vi "ECC_v2.vi"() -> ()   [LabVIEW 2013]
uses:
  state_machine.ctl
  <vilib>/DAQmx/write.llb/DAQmx Write (Analog Wfm 1Chan NSamp).vi
  <vilib>/DAQmx/create/channels.llb/DAQmx Create Channel (AO-Voltage-Basic).vi
  <vilib>/DAQmx/configure/timing.llb/DAQmx Timing (Use Waveform).vi
  <vilib>/DAQmx/miscellaneous.llb/DAQmx Fill In Error Info.vi
panel:
  out "AMP_status":bool
  in  "APS/APM":bool
  in  "AMP address":tag="Dev1/port0/line0"
  in  "R&S/5181":bool=TRUE
  out "Pause, s":i32
  out "APS_off_status":bool=TRUE
  out "R&S_off_status":bool=TRUE
  out "Countdown":u32
  in  "Rep_delay":u32
  in  "Finite/Continuous":bool
  in  "ResumeSweep":bool
  in  "PauseSweep":bool
  in  "RF_off_rep":bool
  in  "RF_off_set":bool
  in  "RF_off_cycle":bool
  in  "APS_off_rep":bool=TRUE
  in  "APS_off_set":bool
  in  "APS_off_cycle":bool
  in  "AbortSweep":bool
  in  "Check APS":bool
  in  "ON/OFF_APS":bool
  in  "Check R&S":bool
  in  "ON/OFF_RF":bool
  in  "Use_APS":bool=TRUE
  out "DAC_status":bool
  out "RF_status":bool
  out "i_Current_repetition":i32
  out "N_Cycles_Created":i32
  out "i_Current_cycle":i32
  in  "M_repetitions":i32 min=0
  in  "Set_of_Cycles":T1(array[cluster])=[{"On/Off"=TRUE, "f0, MHz"=32.5, "fm, kHz"=100, "A, mV"=20, "Waveform"=enum."triangle", "N_steps"=500, "T_sweep, s"=0.1, "N_sweeps"=5, "End_Wait, s"=0}] {"End_Wait, s" step=1; "N_sweeps" min=0 step=1; "T_sweep, s" min=0.0 step=0.001 format="%#_6f"; "N_steps" min=0 step=1; "fm, kHz" step=1; "f0, MHz" min=0.0 step=0.001 format="%#_6f"}
  out "APS_status":bool
  in  "APS address":refnum<visa-resource-name>="COM3"
  in  "Init Devices":bool
  in  "Do Sweep":bool
  in  "Exit":bool
  in  "DAC channel":tag="Dev1/ao0"
  in  "RF address":string(combo)="19"
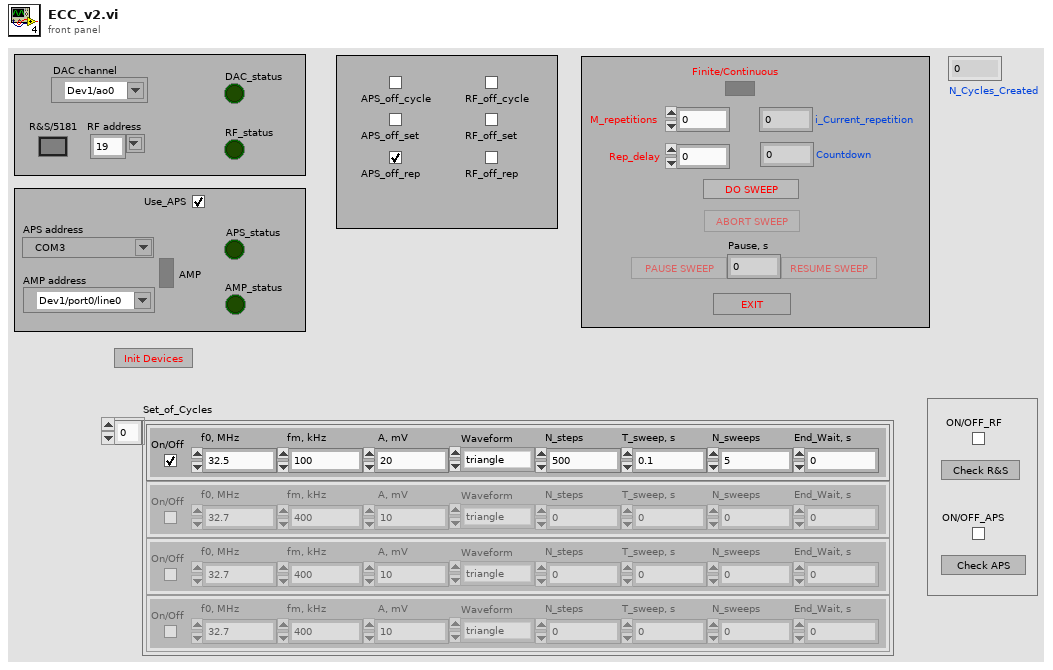
[diagram p1: front panel]
types:
  T1 = cluster{"On/Off":bool, "f0, MHz":dbl, "fm, kHz":i32, "A, mV":i32, "Waveform":enum16{"triangle", "saw_direct", "saw_invert", "sine"}, "N_steps":i32, "T_sweep, s":dbl, "N_sweeps":i32, "End_Wait, s":u32}[]
  T2 = typedef "state_machine.ctl" = enum16{"idle", "init_daq", "init_rf", "init_ps", "cycle_start", "get_wf", "rf_on", "rf_off", "rf_set", "ps_on", "ps_off", "daq_start", "daq_stop", "daq_wait", "daq_dt", "daq_v", "delay", "cycle_reset", "exit", "repetition_reset"}
  T3 = enum8{"Enabled", "Disabled", "Disabled and Grayed Out"}
  T4 = cluster{"On/Off":bool, "f0, MHz":dbl, "fm, kHz":i32, "A, mV":i32, "Waveform":enum16{"triangle", "saw_direct", "saw_invert", "sine"}, "N_steps":i32, "T_sweep, s":dbl, "N_sweeps":i32, "End_Wait, s":u32}
  T5 = enum16{"triangle", "saw_direct", "saw_invert", "sine"}
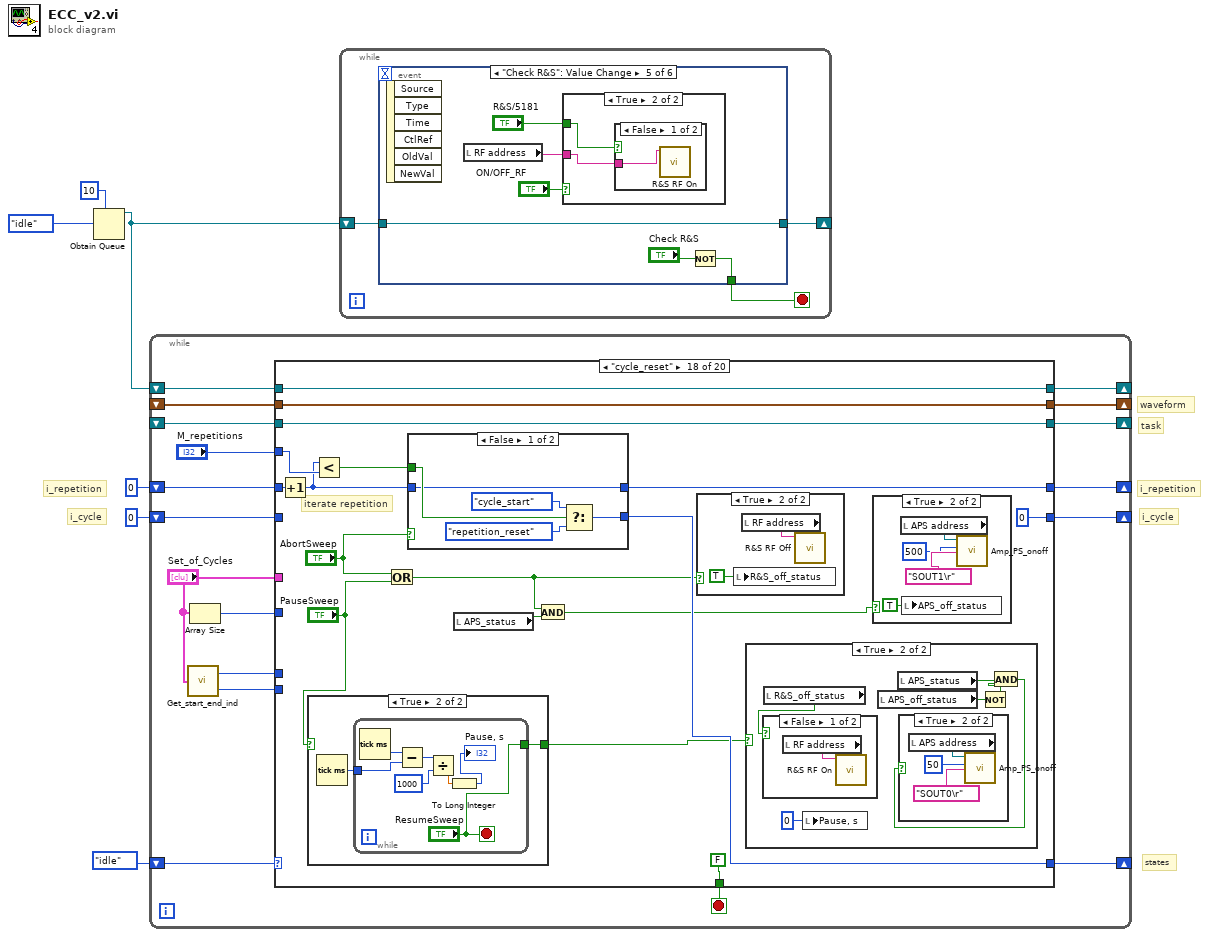
[diagram p0: block diagram]
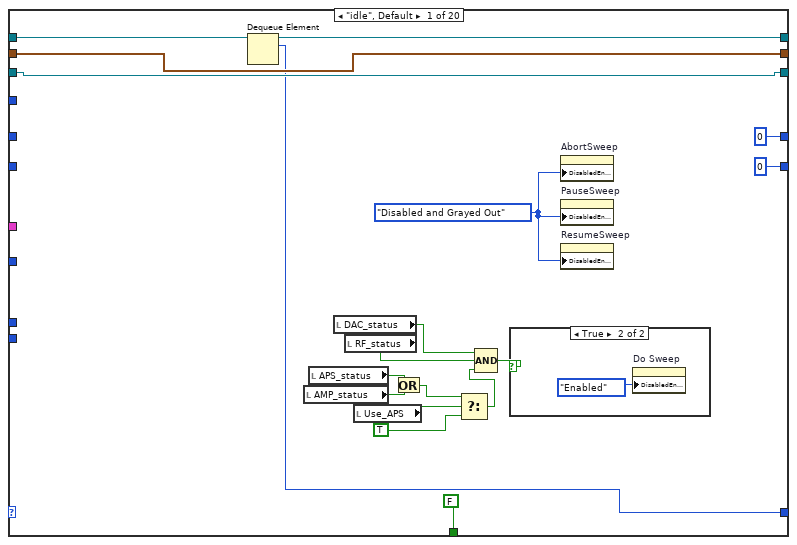
[diagram p2: hidden frame]
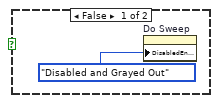
[diagram p3: hidden frame]
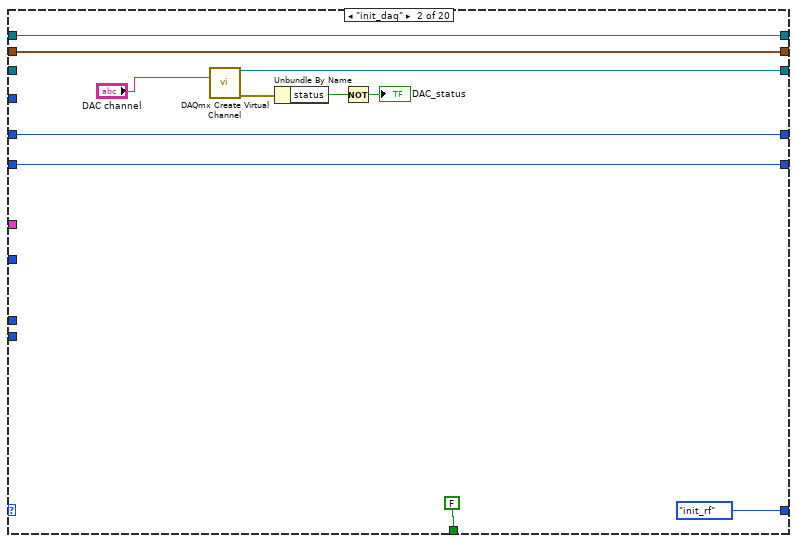
[diagram p4: hidden frame]
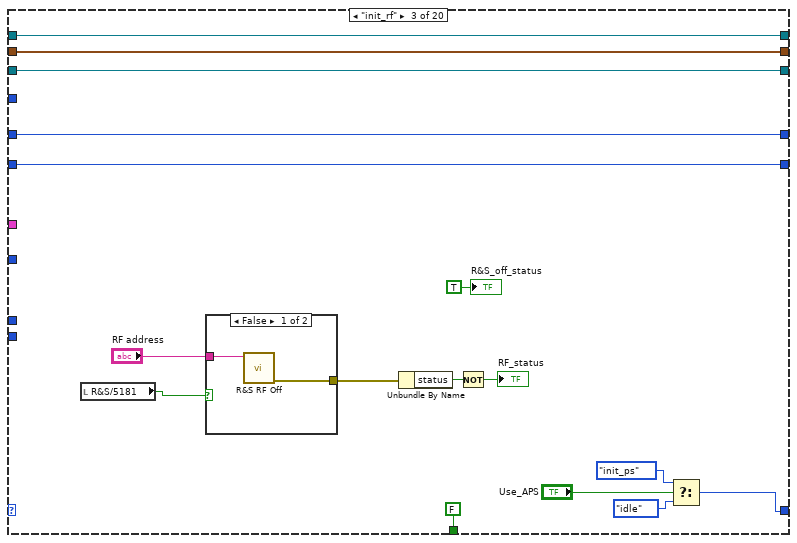
[diagram p5: hidden frame]
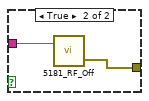
[diagram p6: hidden frame]
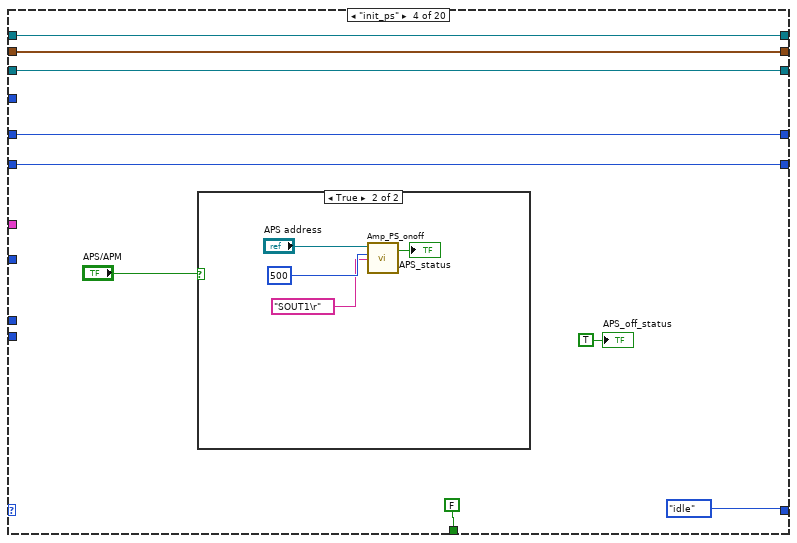
[diagram p7: hidden frame]
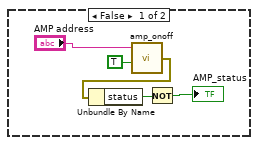
[diagram p8: hidden frame]
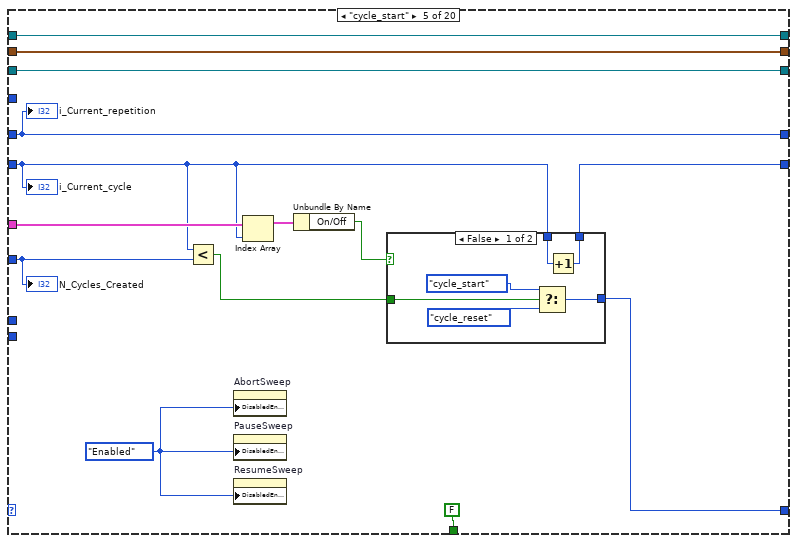
[diagram p9: hidden frame]
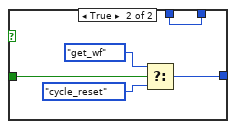
[diagram p10: hidden frame]
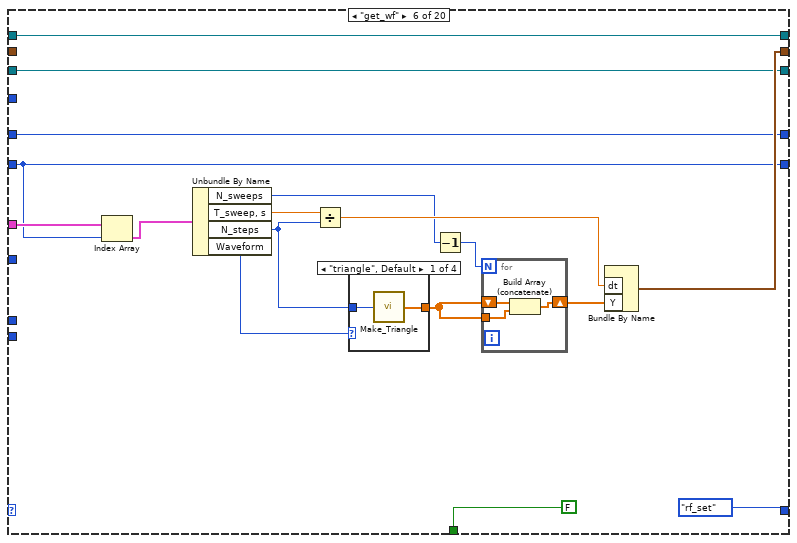
[diagram p11: hidden frame]
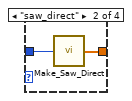
[diagram p12: hidden frame]
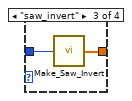
[diagram p13: hidden frame]
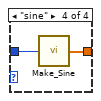
[diagram p14: hidden frame]
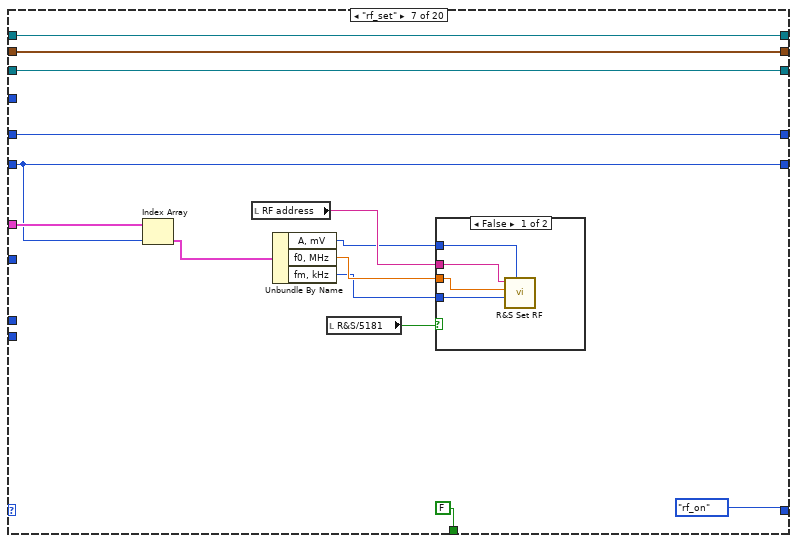
[diagram p15: hidden frame]
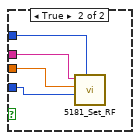
[diagram p16: hidden frame]
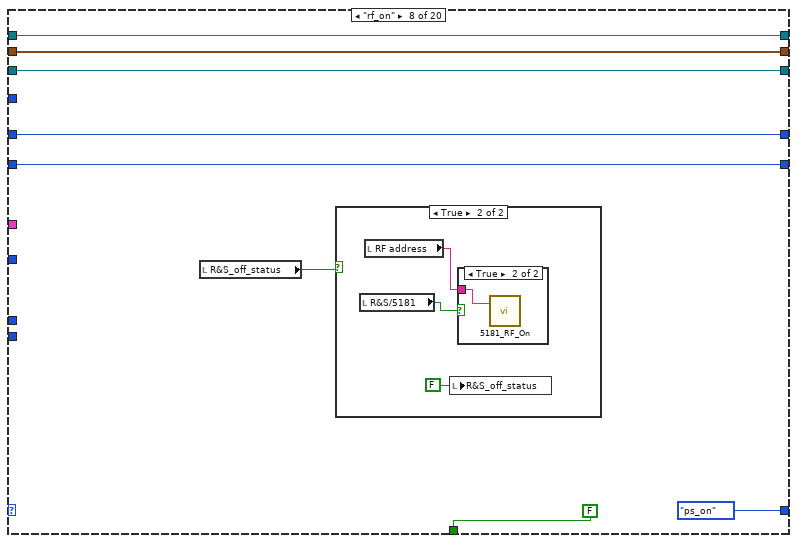
[diagram p17: hidden frame]
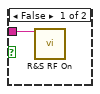
[diagram p19: hidden frame]
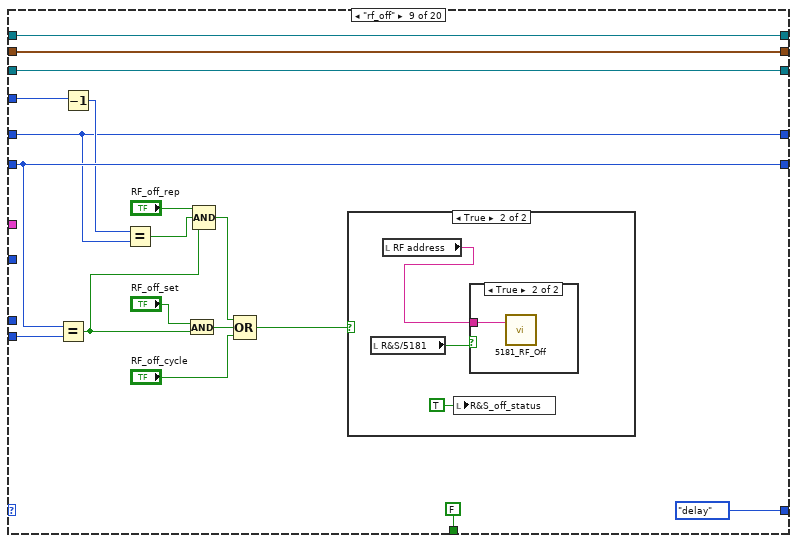
[diagram p20: hidden frame]
diagram:
  # "i_repetition"
  # "i_cycle"
  # "i_repetition"
  # "i_cycle"
  # "states"
  # "waveform"
  # "task"
  n1 = Obtain Queue(max queue size (-1, unlimited)=10, element data type=state_machine."idle") -> (queue out=w4:refnum<queue>)  [unwired: 3 in, 2 out]
  n2 = while {
    shift-right: [w19] -> _
    shift-left: state_machine."idle" -> [w24]
    shift-right: [w23] -> _
    shift-left: _ -> [w21]
    shift-right: [w22] -> _
    shift-left: _ -> [w20]
    shift-right: [w17] -> _
    shift-left: w4 -> [w18]
    shift-right: [w15] -> _
    shift-left: 0 -> [w14]
    shift-right: [w13] -> _
    shift-left: 0 -> [w12]
    stop <- w16 stop-if-true
    n3 = call "Get_start_end_ind.vi"("Set_of_Cycles"="Set_of_Cycles") -> ("start_ind"=w9:i32, "end_ind"=w8:i32)
    n4 = Array Size(array="Set_of_Cycles") -> (size(s)=w11:i32)
    n5 = case shown="\"cycle_reset\"" w24 {
      selector: w24 -> [_ _ _ _ _ _ _ _ _ _ _ _ _ _ _ _ _ _ w376 _]
      tunnel: [w42 w54 w71 w84 w97 w128 w157 w174 w197 w216 w237 w264 w272 w280 w289 w296 w308 w326 w373 w384] -> w23
      tunnel: "Set_of_Cycles" -> [_ _ _ _ w107 w135 w159 _ _ _ _ _ _ _ _ _ w305 _ _ _]
      tunnel: [w41 w53 w70 w83 w98 w129 w156 w175 w198 w215 w236 w263 w271 w279 w288 w297 w309 w325 w372 w385] -> w22
      tunnel: w21 -> [w42 _ w71 w84 w97 w128 w157 w174 w197 w216 w237 w265 w273 w281 w290 w298 w308 w326 w373 w384]
      tunnel: w20 -> [w41 w53 w70 w83 w98 _ w156 w175 w198 w215 w236 w263 w271 w279 w288 w297 w309 w325 w372 w385]
      tunnel: [w38 state_machine."init_rf" w61 state_machine."idle" w103 state_machine."rf_set" state_machine."rf_on" state_machine."ps_on" state_machine."delay" state_machine."daq_dt" state_machine."rf_off" state_machine."daq_wait" state_machine."ps_off" state_machine."daq_stop" state_machine."daq_v" state_machine."daq_start" state_machine."cycle_start" w324 w376 w380] -> w19
      tunnel: w18 -> [w40 w50 w68 w80 w96 w126 w154 w176 w199 w212 w233 w260 w268 w276 w284 w293 w310 w327 w375 w387]
      tunnel: [w39 w50 w68 w80 w96 w126 w154 w176 w199 w212 w233 w260 w268 w276 w284 w293 w310 w327 w375 w387] -> w17
      tunnel: [FALSE FALSE FALSE FALSE FALSE FALSE FALSE FALSE FALSE FALSE FALSE FALSE FALSE FALSE FALSE FALSE FALSE FALSE TRUE FALSE] -> w16
      tunnel: w11 -> [_ _ _ _ w99 _ _ _ _ _ _ _ _ _ _ _ _ _ _ _]
      tunnel: [0 w49 w67 w79 w102 w119 w152 w170 w193 w210 w231 w259 w267 w275 w283 w292 w300 0 w371 w386] -> w15
      tunnel: w14 -> [_ w49 w67 w79 w100 w119 w152 w170 w193 w210 w231 w259 w267 w275 w283 w292 w299 _ w371 w386]
      tunnel: [0 w48 w66 w78 w95 w121 w153 w173 w185 w211 w227 w258 w266 w274 w282 w291 w307 w321 w370 0] -> w13
      tunnel: w12 -> [_ w48 w66 w78 w95 w121 w153 w173 w185 w211 w227 w258 w266 w274 w282 w291 w307 w322 w370 _]
      tunnel: "M_repetitions" -> [_ _ _ _ _ _ _ _ w190 _ w229 _ _ _ _ _ _ w329 _ _]
      tunnel: w9 -> [_ _ _ _ _ _ _ _ _ _ _ _ _ _ _ _ _ _ _ _]
      tunnel: w8 -> [_ _ _ _ _ _ _ _ w194 _ w232 _ _ _ _ _ _ _ _ _]
      frame "idle", Default {
        w28 = T3."Disabled and Grayed Out" ("Disabled")
        n6 = Dequeue Element(queue=w40) -> (queue out=w39:refnum<queue>, element=w38:T2)  [unwired: 2 in, 2 out]
        n7 = local read "AMP_status"() -> (w26:bool)
        n8 = local read "APS_status"() -> (w27:bool)
        n9 = local read "DAC_status"() -> (w34:bool)
        n10 = local read "RF_status"() -> (w33:bool)
        n11 = local read "Use_APS"() -> (w32:bool)
        n12 = Or(x=w27, y=w26) -> (x .or. y?=w25:bool)
        n13 = Select(t=w25, s=w32, f=TRUE) -> (s? t:f=w30:bool)
        n14 = Compound Arithmetic op=AND(w34, w33, w30) -> (w29:bool)
        n15 = case shown="True" w29 {
          frame False {
            n16 = property on="Do Sweep" class="Bool"("DisabledEnum"=T3."Disabled and Grayed Out" ("Disabled")) -> ()  [unwired: 2 in, 2 out]
          }
          frame True {
            n17 = property on="Do Sweep" class="Bool"("DisabledEnum"=T3."Enabled" ("Disabled")) -> ()  [unwired: 2 in, 2 out]
          }
        }
        n18 = property on="AbortSweep" class="Bool"("DisabledEnum"=w28) -> ()  [unwired: 2 in, 2 out]
        n19 = property on="PauseSweep" class="Bool"("DisabledEnum"=w28) -> ()  [unwired: 2 in, 2 out]
        n20 = property on="ResumeSweep" class="Bool"("DisabledEnum"=w28) -> ()  [unwired: 2 in, 2 out]
      }
      frame "init_daq" {
        n21 = call-poly <vilib>:"DAQmx Create Virtual Channel.vi"("physical channels"="DAC channel") -> ("task out"=w54:refnum<k21>, "error out"=w47:errorcluster)  [unwired: 13 in]
        n22 = Unbundle By Name(w47) -> ("status"=w46:bool)
        n23 = Not(x=w46) -> (.not. x?=→"DAC_status":bool)
      }
      frame "init_rf" {
        n24 = local read "R&S/5181"() -> (w56:bool)
        n25 = case shown="False" w56 {
          tunnel: "RF address" -> [w73 w75]
          tunnel: [w72 w74] -> w57
          frame False {
            n26 = call "R&S RF Off.vi"("address"=w73) -> ("error out"=w72:errorcluster)  [unwired: 5 in, 1 out]
          }
          frame True {
            n27 = call "5181_RF_Off.vi"("address"=w75) -> ("error out"=w74:errorcluster)  [unwired: 1 in, 1 out]
          }
        }
        n28 = Unbundle By Name(w57) -> ("status"=w64:bool)
        n29 = Not(x=w64) -> (.not. x?=→"RF_status":bool)
        n30 = Select(t=state_machine."init_ps", s="Use_APS", f=state_machine."idle") -> (s? t:f=w61:T2)
        "R&S_off_status" <- TRUE ("R&S_off_status")
      }
      frame "init_ps" {
        n31 = case shown="True" "APS/APM" {
          frame False {
            n32 = call "amp_onoff.vi"("amp_onoff"=TRUE, "AMP address"="AMP address") -> ("error out"=w87:errorcluster)  [unwired: 1 in]
            n33 = Unbundle By Name(w87) -> ("status"=w88:bool)
            n34 = Not(x=w88) -> (.not. x?=→"AMP_status":bool)
          }
          frame True {
            n35 = call "Amp_PS_onoff.vi"("On/Off Control"="SOUT1\r", "delay before read (ms)"=u32 500, "Amp PS address"="APS address") -> ("status"=→"APS_status":bool)  [unwired: 1 in, 1 out]
          }
        }
        "APS_off_status" <- TRUE ("APS_off_status")
      }
      frame "cycle_start" {
        w94 = T3."Enabled" ("Disabled")
        n36 = Less?(x=w100, y=w99) -> (x < y?=w104:bool)
        n37 = property on="AbortSweep" class="Bool"("DisabledEnum"=w94) -> ()  [unwired: 2 in, 2 out]
        n38 = property on="PauseSweep" class="Bool"("DisabledEnum"=w94) -> ()  [unwired: 2 in, 2 out]
        n39 = property on="ResumeSweep" class="Bool"("DisabledEnum"=w94) -> ()  [unwired: 2 in, 2 out]
        n40 = Index Array(array=w107, index=w100) -> (element=w106:T4)
        n41 = Unbundle By Name(w106) -> ("On/Off"=w105:bool)
        n42 = case shown="False" w105 {
          tunnel: w104 -> [w111 w117]
          tunnel: [w108 w116] -> w103
          tunnel: w100 -> [w113 w114]
          tunnel: [w112 w114] -> w102
          frame False {
            n43 = Select(t=state_machine."cycle_start", s=w111, f=state_machine."cycle_reset") -> (s? t:f=w108:T2)
            n44 = Increment(x=w113) -> (x+1=w112:i32)
          }
          frame True {
            n45 = Select(t=state_machine."get_wf", s=w117, f=state_machine."cycle_reset") -> (s? t:f=w116:T2)
          }
        }
        "N_Cycles_Created" <- w99
        "i_Current_cycle" <- w100
        "i_Current_repetition" <- w95
      }
      frame "get_wf" {
        n46 = Index Array(array=w135, index=w119) -> (element=w134:T4)
        n47 = Unbundle By Name(w134) -> ("N_sweeps"=w125:i32, "T_sweep, s"=w123:dbl, "N_steps"=w122:i32, "Waveform"=w124:T5)
        n48 = Divide(x=w123, y=w122) -> (x/y=w131:dbl)
        n49 = case shown="\"triangle\", Default" w124 {
          tunnel: w122 -> [w140 w142 w144 w146]
          tunnel: [w139 w141 w143 w145] -> w132
          frame "triangle", Default {
            n50 = call "Make_Triangle.vi"("N_steps_1"=w140) -> ("TriangleWaveform"=w139:dbl[])
          }
          frame "saw_direct" {
            n51 = call "Make_Saw_Direct.vi"("N_steps_1"=w142) -> ("SawDirectWaveform"=w141:dbl[])
          }
          frame "saw_invert" {
            n52 = call "Make_Saw_Invert.vi"("N_steps_1"=w144) -> ("SawInvertWaveform"=w143:dbl[])
          }
          frame "sine" {
            n53 = call "Make_Sine.vi"("N_steps_1"=w146) -> ("SineWaveform"=w145:dbl[])
          }
        }
        n54 = Decrement(x=w125) -> (x-1=w130:i32)
        n55 = for {
          N: w130 -> [_]
          shift-right: [w136] -> w133
          shift-left: w132 -> [w138]
          tunnel: w132 -> [w137]
          n56 = Build Array (concatenate)(w138, w137) -> (w136:dbl[])
        }
        n57 = Bundle By Name("dt"=w131, "Y"=w133) -> (w129:waveform(dbl))  [unwired: 1 in]
      }
      frame "rf_set" {
        n58 = Index Array(array=w159, index=w152) -> (element=w158:T4)
        n59 = local read "RF address"() -> (w160:string)
        n60 = Unbundle By Name(w158) -> ("A, mV"=w151:i32, "f0, MHz"=w150:dbl, "fm, kHz"=w149:i32)
        n61 = local read "R&S/5181"() -> (w147:bool)
        n62 = case shown="False" w147 {
          tunnel: w160 -> [w164 w168]
          tunnel: w151 -> [w163 w167]
          tunnel: w150 -> [w162 w166]
          tunnel: w149 -> [w161 w165]
          frame False {
            n63 = call "R&S Set RF.vi"("amplitude (mV)"=w163, "modulation (kHz)"=w161, "center frequency (MHz)"=w162, "address"=w164) -> ()  [unwired: 3 in, 2 out]
          }
          frame True {
            n64 = call "5181_Set_RF.vi"("address"=w168, "center frequency (MHz)"=w166, "modulation (kHz)"=w165, "amplitude (mV)"=w167) -> ()  [unwired: 1 in, 2 out]
          }
        }
      }
      frame "rf_on" {
        n65 = local read "R&S_off_status"() -> (w169:bool)
        n66 = case shown="True" w169 {
          frame False {
          }
          frame True {
            n67 = local read "R&S/5181"() -> (w177:bool)
            n68 = local read "RF address"() -> (w179:string)
            n69 = local write "R&S_off_status"(FALSE ("R&S_off_status")) -> ()
            n70 = case shown="True" w177 {
              tunnel: w179 -> [w180 w181]
              frame False {
                n71 = call "R&S RF On.vi"("address"=w180) -> ()  [unwired: 5 in, 2 out]
              }
              frame True {
                n72 = call "5181_RF_On.vi"("address"=w181) -> ()  [unwired: 1 in, 2 out]
              }
            }
          }
        }
      }
      frame "rf_off" {
        n73 = Equal?(x=w193, y=w194) -> (x = y?=w182:bool)
        n74 = Decrement(x=w190) -> (x-1=w186:i32)
        n75 = Equal?(x=w186, y=w185) -> (x = y?=w183:bool)
        n76 = And(x="RF_off_set", y=w182) -> (x .and. y?=w189:bool)
        n77 = Compound Arithmetic op=AND("RF_off_rep", w183, w182) -> (w187:bool)
        n78 = Compound Arithmetic op=OR(w187, w189, "RF_off_cycle") -> (w191:bool)
        n79 = case shown="True" w191 {
          frame False {
          }
          frame True {
            n80 = local read "R&S/5181"() -> (w200:bool)
            n81 = local read "RF address"() -> (w202:string)
            n82 = local write "R&S_off_status"(TRUE ("R&S_off_status")) -> ()
            n83 = case shown="True" w200 {
              tunnel: w202 -> [w203 w204]
              frame False {
                n84 = call "R&S RF Off.vi"("address"=w203) -> ()  [unwired: 5 in, 2 out]
              }
              frame True {
                n85 = call "5181_RF_Off.vi"("address"=w204) -> ()  [unwired: 1 in, 2 out]
              }
            }
          }
        }
      }
      frame "ps_on" {
        n86 = local read "APS_status"() -> (w205:bool)
        n87 = local read "APS_status"() -> (w207:bool)
        n88 = local read "APS_off_status"() -> (w209:bool)
        n89 = Or(x=w207, y=w205) -> (x .or. y?=w206:bool)
        n90 = And(x=w206, y=w209) -> (x .and. y?=w208:bool)
        n91 = case shown="True" w208 {
          frame False {
          }
          frame True {
            n92 = local read "APS/APM"() -> (w217:bool)
            n93 = case shown="True" w217 {
              frame False {
                n94 = local read "AMP address"() -> (w219:tag)
                n95 = call "amp_onoff.vi"("amp_onoff"=TRUE, "AMP address"=w219) -> ()  [unwired: 1 in, 1 out]
              }
              frame True {
                n96 = local read "APS address"() -> (w221:refnum<visa-resource-name>)
                n97 = call "Amp_PS_onoff.vi"("On/Off Control"="SOUT0\r", "delay before read (ms)"=u32 500, "Amp PS address"=w221) -> ()  [unwired: 1 in, 2 out]
              }
            }
            n98 = local write "APS_off_status"(FALSE ("APS_off_status")) -> ()
          }
        }
      }
      frame "ps_off" {
        n99 = Decrement(x=w229) -> (x-1=w228:i32)
        n100 = local read "APS_status"() -> (w225:bool)
        n101 = local read "APS_status"() -> (w226:bool)
        n102 = Or(x=w226, y=w225) -> (x .or. y?=w224:bool)
        n103 = case shown="True" w224 {
          selector: w224 -> [w238 _]
          tunnel: w232 -> [_ w250]
          tunnel: w231 -> [_ w249]
          tunnel: [w238 w244] -> w230
          tunnel: w228 -> [_ w240]
          tunnel: w227 -> [_ w241]
          frame False {
          }
          frame True {
            n104 = Equal?(x=w240, y=w241) -> (x = y?=w246:bool)
            n105 = Equal?(x=w249, y=w250) -> (x = y?=w239:bool)
            n106 = Compound Arithmetic op=AND("APS_off_rep", w246, w239) -> (w243:bool)
            n107 = And(x="APS_off_set", y=w239) -> (x .and. y?=w245:bool)
            n108 = Compound Arithmetic op=OR(w243, w245, "APS_off_cycle") -> (w244:bool)
          }
        }
        n109 = case shown="True" w230 {
          frame False {
          }
          frame True {
            n110 = local read "APS/APM"() -> (w251:bool)
            n111 = case shown="True" w251 {
              frame False {
                n112 = local read "AMP address"() -> (w253:tag)
                n113 = call "amp_onoff.vi"("amp_onoff"=FALSE, "AMP address"=w253) -> ()  [unwired: 1 in, 1 out]
              }
              frame True {
                n114 = local read "APS address"() -> (w255:refnum<visa-resource-name>)
                n115 = call "Amp_PS_onoff.vi"("On/Off Control"="SOUT1\r", "delay before read (ms)"=u32 500, "Amp PS address"=w255) -> ()  [unwired: 1 in, 2 out]
              }
            }
            n116 = local write "APS_off_status"(TRUE ("APS_off_status")) -> ()
          }
        }
      }
      frame "daq_start" {
        n117 = call <vilib>:"DAQmx Start Task.vi"("task/channels in"=w265) -> ("task out"=w264:refnum<k21>)  [unwired: 13 in, 1 out]
      }
      frame "daq_stop" {
        n118 = call <vilib>:"DAQmx Stop Task.vi"("task/channels in"=w273) -> ("task out"=w272:refnum<k21>)  [unwired: 13 in, 1 out]
      }
      frame "daq_wait" {
        n119 = call <vilib>:"DAQmx Wait Until Done.vi"("task/channels in"=w281) -> ("task out"=w280:refnum<k21>)  [unwired: 13 in, 1 out]
      }
      frame "daq_dt" {
        w287 = 10178 items=["Finite Samples"=10178, "Continuous Samples"=10123, "Hardware Timed Single Point"=12522] ("sample mode")
        n120 = call-poly <vilib>:"DAQmx Timing.vi"("task/channels in"=w290, "sample mode"=w287, "waveform"=w288) -> ("task out"=w289:refnum<k21>)  [unwired: 11 in, 1 out]
      }
      frame "daq_v" {
        n121 = call-poly <vilib>:"DAQmx Write.vi"("task/channels in"=w298, "data"=w297) -> ("task out"=w296:refnum<k21>)  [unwired: 11 in, 2 out]
      }
      frame "delay" {
        # "iterate cycle"
        n122 = Increment(x=w299) -> (x+1=w300:i32)
        n123 = Index Array(array=w305, index=w299) -> (element=w306:T4)
        n124 = Unbundle By Name(w306) -> ("End_Wait, s"=w303:u32)
        n125 = Equal To 0?(x=w303) -> (x = 0?=w304:bool)
        n126 = case shown="True" w304 {
          tunnel: w303 -> [w311 _]
          frame False {
            n127 = Multiply(x=u32 1000 ("y"), y=w311) -> (x*y=w313:u32)
            n128 = Wait (ms)(milliseconds to wait=w313) -> ()  [unwired: 1 out]
          }
          frame True {
          }
        }
      }
      frame "cycle_reset" {
        # "iterate repetition"
        n129 = Increment(x=w322) -> (x+1=w314:i32)
        n130 = case shown="True" "PauseSweep" {
          selector: "PauseSweep" -> [w341 _]
          tunnel: [w341 w342] -> w318
          frame False {
          }
          frame True {
            n131 = Tick Count (ms)() -> (millisecond timer value=w343:u32)
            n132 = while {
              tunnel: w343 -> [w349]
              tunnel: ["ResumeSweep"] -> w342
              stop <- "ResumeSweep" stop-if-true
              n133 = Tick Count (ms)() -> (millisecond timer value=w350:u32)
              n134 = Subtract(x=w350, y=w349) -> (x-y=w348:u32)
              n135 = Divide(x=w348, y=u32 1000) -> (x/y=w346:dbl)
              n136 = To Long Integer(number=w346) -> (32bit integer=→"Pause, s":i32)
            }
          }
        }
        n137 = Less?(x=w314, y=w329) -> (x < y?=w323:bool)
        n138 = Or(x="AbortSweep", y="PauseSweep") -> (x .or. y?=w315:bool)
        n139 = case shown="False" "AbortSweep" {
          tunnel: [w359 state_machine."idle"] -> w324
          tunnel: w323 -> [w358 _]
          tunnel: w314 -> [w357 _]
          tunnel: [w357 0] -> w321
          frame False {
            n140 = Select(t=state_machine."cycle_start", s=w358, f=state_machine."repetition_reset") -> (s? t:f=w359:T2)
          }
          frame True {
            w363 = T3."Enabled" ("Disabled")
            n141 = property on="Check APS" class="Bool"("DisabledEnum"=w363) -> ()  [unwired: 2 in, 2 out]
            n142 = property on="Check R&S" class="Bool"("DisabledEnum"=w363) -> ()  [unwired: 2 in, 2 out]
          }
        }
        n143 = local read "APS_status"() -> (w316:bool)
        n144 = And(x=w315, y=w316) -> (x .and. y?=w317:bool)
        n145 = case shown="True" w315 {
          frame False {
          }
          frame True {
            n146 = local write "R&S_off_status"(TRUE ("R&S_off_status")) -> ()
            n147 = local read "RF address"() -> (w352:string)
            n148 = call "R&S RF Off.vi"("address"=w352) -> ()  [unwired: 5 in, 2 out]
          }
        }
        n149 = case shown="True" w318 {
          frame False {
          }
          frame True {
            n150 = local read "R&S_off_status"() -> (w336:bool)
            n151 = case shown="False" w336 {
              frame False {
                n152 = local read "RF address"() -> (w340:string)
                n153 = call "R&S RF On.vi"("address"=w340) -> ()  [unwired: 5 in, 2 out]
              }
              frame True {
              }
            }
            n154 = local write "Pause, s"(0 ("Pause, s")) -> ()
            n155 = local read "APS_off_status"() -> (w334:bool)
            n156 = local read "APS_status"() -> (w335:bool)
            n157 = Not(x=w334) -> (.not. x?=w333:bool)
            n158 = And(x=w335, y=w333) -> (x .and. y?=w332:bool)
            n159 = case shown="True" w332 {
              frame False {
              }
              frame True {
                n160 = local read "APS address"() -> (w337:refnum<visa-resource-name>)
                n161 = call "Amp_PS_onoff.vi"("On/Off Control"="SOUT0\r", "delay before read (ms)"=u32 50, "Amp PS address"=w337) -> ()  [unwired: 1 in, 2 out]
              }
            }
          }
        }
        n162 = case shown="True" w317 {
          frame False {
          }
          frame True {
            n163 = local read "APS address"() -> (w354:refnum<visa-resource-name>)
            n164 = local write "APS_off_status"(TRUE ("APS_off_status")) -> ()
            n165 = call "Amp_PS_onoff.vi"("On/Off Control"="SOUT1\r", "delay before read (ms)"=u32 500, "Amp PS address"=w354) -> ()  [unwired: 1 in, 2 out]
          }
        }
      }
      frame "exit" {
        w365 = FALSE ("DAC_status")
        n166 = local read "APS address"() -> (w368:refnum<visa-resource-name>)
        n167 = local read "Use_APS"() -> (w369:bool)
        n168 = local read "RF address"() -> (w367:string)
        n169 = case shown="False" w369 {
          tunnel: w368 -> [_ w377]
          frame False {
          }
          frame True {
            n170 = call "Amp_PS_onoff.vi"("On/Off Control"="SOUT1\r", "delay before read (ms)"=u32 50, "Amp PS address"=w377) -> ()  [unwired: 1 in, 2 out]
          }
        }
        n171 = call "R&S RF Off.vi"("address"=w367) -> ()  [unwired: 5 in, 2 out]
        n172 = property on="Init Devices" class="Bool"("DisabledEnum"=T3."Enabled" ("Disabled")) -> ()  [unwired: 2 in, 2 out]
        n173 = local write "DAC_status"(w365) -> ()
        n174 = local write "RF_status"(w365) -> ()
        n175 = local write "APS_status"(w365) -> ()
      }
      frame "repetition_reset" {
        n176 = case shown="True" "Finite/Continuous" {
          tunnel: [state_machine."idle" state_machine."cycle_start"] -> w380
          frame False {
          }
          frame True {
            n177 = Tick Count (ms)() -> (millisecond timer value=w390:u32)
            n178 = while {
              tunnel: w390 -> [w397]
              tunnel: "Rep_delay" -> [w393]
              stop <- w395 stop-if-true
              w392 = u32 1000 ("y")
              n179 = Tick Count (ms)() -> (millisecond timer value=w398:u32)
              n180 = Subtract(x=w398, y=w397) -> (x-y=w399:u32)
              n181 = Divide(x=w399, y=w392) -> (x/y=w400:dbl)
              n182 = Wait (ms)(milliseconds to wait=w392) -> ()  [unwired: 1 out]
              n183 = To Long Integer(number=w400) -> (32bit integer=w394:i32)
              n184 = Subtract(x=w393, y=w394) -> (x-y=w396:u32)
              "Countdown" <- w396
              n185 = Less Or Equal To 0?(x=w396) -> (x <= 0?=w395:bool)
            }
          }
        }
      }
    }
  }
  n186 = while {
    shift-right: [w401] -> _
    shift-left: w4 -> [w402]
    stop <- w403 stop-if-true
    n187 = event shown="[4] \"Check R&S\": Value Change" {
      selector: _ -> [_ _ _ _ _ _]
      dyn-events: _ -> [_ _ _ _ _ _]
      timeout: _ -> [_ _ _ _ _ _]
      tunnel: [_ "Exit" w413 w419 w426 w439] -> w403
      tunnel: w402 -> [w404 w407 w412 w418 w423 w436]
      tunnel: [w404 w406 w411 w417 w423 w436] -> w401
      event Timeout {
        n188 = event-data() -> ()  [unwired: 1 in, 3 out]
      }
      event "Exit": Value Change {
        n189 = event-data() -> ()  [unwired: 1 in, 6 out]
        n190 = Enqueue Element(queue=w407, element=state_machine."exit") -> (queue out=w406:refnum<queue>)  [unwired: 2 in, 2 out]
      }
      event "Init Devices": Value Change {
        n191 = event-data() -> ()  [unwired: 1 in, 6 out]
        n192 = Enqueue Element(queue=w412, element=state_machine."init_daq") -> (queue out=w411:refnum<queue>)  [unwired: 2 in, 2 out]
        n193 = property on="Init Devices" class="Bool"("DisabledEnum"=T3."Disabled and Grayed Out" ("Disabled")) -> ()  [unwired: 2 in, 2 out]
        n194 = Not(x="Init Devices") -> (.not. x?=w413:bool)
      }
      event "Do Sweep": Value Change {
        w415 = T3."Disabled and Grayed Out" ("Disabled")
        n195 = event-data() -> ()  [unwired: 1 in, 6 out]
        n196 = Enqueue Element(queue=w418, element=state_machine."cycle_start") -> (queue out=w417:refnum<queue>)  [unwired: 2 in, 2 out]
        n197 = Not(x="Do Sweep") -> (.not. x?=w419:bool)
        n198 = property on="Check R&S" class="Bool"("DisabledEnum"=w415) -> ()  [unwired: 2 in, 2 out]
        n199 = property on="Check APS" class="Bool"("DisabledEnum"=w415) -> ()  [unwired: 2 in, 2 out]
      }
      event "Check R&S": Value Change {
        n200 = event-data() -> ()  [unwired: 1 in, 6 out]
        n201 = local read "RF address"() -> (w424:string)
        n202 = case shown="True" "ON/OFF_RF" {
          tunnel: w424 -> [w428 w432]
          tunnel: "R&S/5181" -> [w427 w431]
          frame False {
            n203 = case shown="True" w427 {
              tunnel: w428 -> [w429 w430]
              frame False {
                n204 = call "R&S RF Off.vi"("address"=w429) -> ()  [unwired: 5 in, 2 out]
              }
              frame True {
                n205 = call "5181_RF_Off.vi"("address"=w430) -> ()  [unwired: 1 in, 2 out]
              }
            }
          }
          frame True {
            n206 = case shown="False" w431 {
              tunnel: w432 -> [w433 w434]
              frame False {
                n207 = call "R&S RF On.vi"("address"=w433) -> ()  [unwired: 5 in, 2 out]
              }
              frame True {
                n208 = call "5181_RF_On.vi"("address"=w434) -> ()  [unwired: 1 in, 2 out]
              }
            }
          }
        }
        n209 = Not(x="Check R&S") -> (.not. x?=w426:bool)
      }
      event "Check APS": Value Change {
        n210 = event-data() -> ()  [unwired: 1 in, 6 out]
        n211 = local read "APS address"() -> (w437:refnum<visa-resource-name>)
        n212 = case shown="False" "ON/OFF_APS" {
          tunnel: w437 -> [w440 w443]
          frame False {
            n213 = call "Amp_PS_onoff.vi"("On/Off Control"="SOUT1\r", "delay before read (ms)"=u32 50, "Amp PS address"=w440) -> ()  [unwired: 1 in, 2 out]
          }
          frame True {
            n214 = call "Amp_PS_onoff.vi"("On/Off Control"="SOUT0\r", "delay before read (ms)"=u32 50, "Amp PS address"=w443) -> ()  [unwired: 1 in, 2 out]
          }
        }
        n215 = Not(x="Check APS") -> (.not. x?=w439:bool)
      }
    }
  }
